vi "Teleop_Flywheel.vi"(11 "Joystick_IN":T1={"Pilot Left Joystick X"=0.015748031496062992, "Pilot Left Joystick Y"=-0.0, "Pilot A Button"=FALSE, "Pilot B Button"=FALSE, "Pilot X Button"=FALSE, "Pilot Y Button"=FALSE, "Pilot Left Bumper"=FALSE, "Pilot Right Bumper"=FALSE, "Pilot View Button"=FALSE, "Pilot Menu Button"=FALSE, "Pilot Left Joystick Press"=FALSE, "Pilot Right Joystick Press"=FALSE, "Pilot Left Trigger"=0.0, "Pilot Right Joystick X"=0.03937007874015748, "Pilot Right Joystick Y"=-0.015748031496062992, "Pilot Right Trigger"=0.0, "Copilot Left Joystick X"=0.0, "Copilot Left Joystick Y"=0.0, "Copilot A Button"=FALSE, "Copilot B Button"=FALSE, "Copilot X Button"=FALSE, "Copilot Y Button"=FALSE, "Copilot Left Bumper"=FALSE, "Copilot Right Bumper"=FALSE, "Copilot View Button"=FALSE, "Copilot Menu Button"=FALSE, "Copilot Left Joystick Press"=FALSE, "Copilot Right Joystick Press"=FALSE, "Copilot Left Trigger"=0.0, "Copilot Right Joystick X"=0.0, "Copilot Right Joystick Y"=0.0, "Copilot Right Trigger"=0.0, "Pilot D-pad North"=FALSE, "Pilot D-pad South"=FALSE, "Pilot D-pad East"=FALSE, "Pilot D-pad West"=FALSE, "Pilot D-pad NE "=FALSE, "Pilot D-pad SE"=FALSE, "Pilot D-pad SW"=FALSE, "Pilot D-pad NW"=FALSE, "CoPilot D-pad North"=TRUE, "CoPilot D-pad South"=FALSE, "CoPilot D-pad East"=FALSE, "CoPilot D-pad West"=FALSE, "CoPilot D-pad NE"=FALSE, "CoPilot D-pad SE"=FALSE, "CoPilot D-pad SW"=FALSE, "CoPilot D-pad NW"=FALSE, "Pilot Left Trigger Pressed"=FALSE, "Pilot Right Trigger Pressed"=FALSE, "CoPilot Left Trigger Pressed"=FALSE, "CoPilot Right Trigger Pressed"=FALSE}) -> ()   [LabVIEW 2019]
uses:
  Utility_VIs/Joystick_Controls.ctl
  Globals/Flywheel_Globals.vi
  Subsystems/Flywheel/Flywheel_States.ctl
  Subsystems/Flywheel/Flywheel_Cluster.ctl
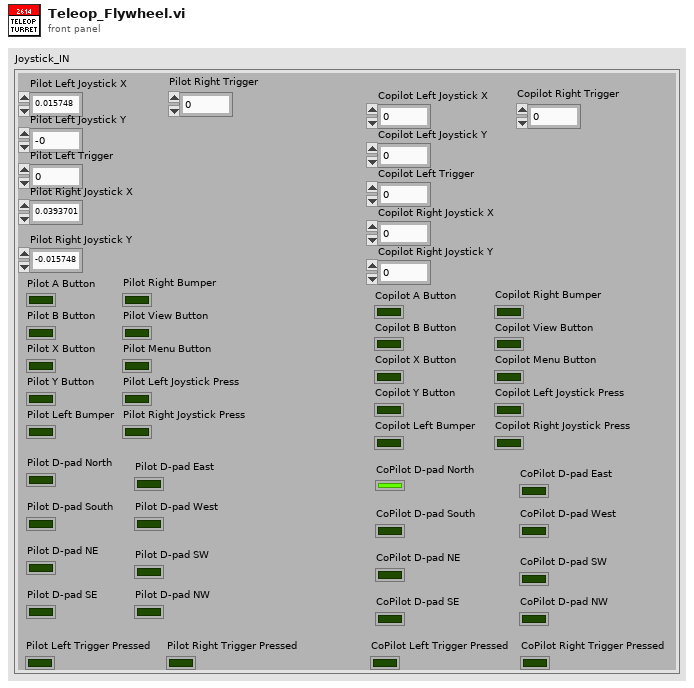
[diagram p1: front panel]
types:
  T1 = typedef "Joystick_Controls.ctl" = cluster{"Pilot Left Joystick X":dbl, "Pilot Left Joystick Y":dbl, "Pilot A Button":bool, "Pilot B Button":bool, "Pilot X Button":bool, "Pilot Y Button":bool, "Pilot Left Bumper":bool, "Pilot Right Bumper":bool, "Pilot View Button":bool, "Pilot Menu Button":bool, "Pilot Left Joystick Press":bool, "Pilot Right Joystick Press":bool, "Pilot Left Trigger":dbl, "Pilot Right Joystick X":dbl, "Pilot Right Joystick Y":dbl, "Pilot Right Trigger":dbl, "Copilot Left Joystick X":dbl, "Copilot Left Joystick Y":dbl, "Copilot A Button":bool, "Copilot B Button":bool, "Copilot X Button":bool, "Copilot Y Button":bool, "Copilot Left Bumper":bool, "Copilot Right Bumper":bool, "Copilot View Button":bool, "Copilot Menu Button":bool, "Copilot Left Joystick Press":bool, "Copilot Right Joystick Press":bool, "Copilot Left Trigger":dbl, "Copilot Right Joystick X":dbl, "Copilot Right Joystick Y":dbl, "Copilot Right Trigger":dbl, "Pilot D-pad North":bool, "Pilot D-pad South":bool, "Pilot D-pad East":bool, "Pilot D-pad West":bool, "Pilot D-pad NE ":bool, "Pilot D-pad SE":bool, "Pilot D-pad SW":bool, "Pilot D-pad NW":bool, "CoPilot D-pad North":bool, "CoPilot D-pad South":bool, "CoPilot D-pad East":bool, "CoPilot D-pad West":bool, "CoPilot D-pad NE":bool, "CoPilot D-pad SE":bool, "CoPilot D-pad SW":bool, "CoPilot D-pad NW":bool, "Pilot Left Trigger Pressed":bool, "Pilot Right Trigger Pressed":bool, "CoPilot Left Trigger Pressed":bool, "CoPilot Right Trigger Pressed":bool}
  T2 = typedef "Flywheel_Cluster.ctl" = cluster{"Flywheel_Throttle":dbl, "Control_States":T3, "Auto_Speed":bool, "Flywheel_On":bool}
  T3 = typedef "Flywheel_States.ctl" = enum16{"No-Op", "Percent_Voltage", "Speed_Control_Manual", "Speed_Control_Auto"}
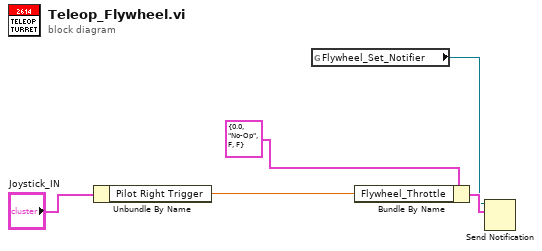
[diagram p0: block diagram]
diagram:
  n1 = Unbundle By Name("Joystick_IN") -> ("Pilot Right Trigger"=w1:dbl)
  n2 = global read "Flywheel_Globals.vi" "Flywheel_Set_Notifier"() -> (w3:refnum<notifier>)
  n3 = Bundle By Name(cluster=T2 {"Flywheel_Throttle"=0.0, "Control_States"=enum."No-Op", "Auto_Speed"=FALSE, "Flywheel_On"=FALSE} ("Flywheel_Cluster"), "Flywheel_Throttle"=w1) -> (w4:T2)
  n4 = Send Notification(notification=w4, notifier=w3) -> ()  [unwired: 1 in, 2 out]
